vi "VariablesToString_Array.vi"(3 "Format":string="%0.2f", 4 "Terminate?":bool=TRUE, 5 "ValueIn":dbl[](array[numeric]), 6 "FieldName":string, 7 "Type":enum16{"Normal", "Matlab"}(ring)) -> (1 "StringOut":string)   [LabVIEW 2013]
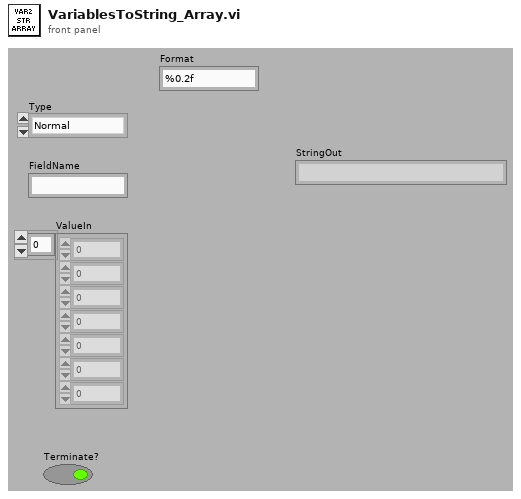
[diagram p1: front panel]
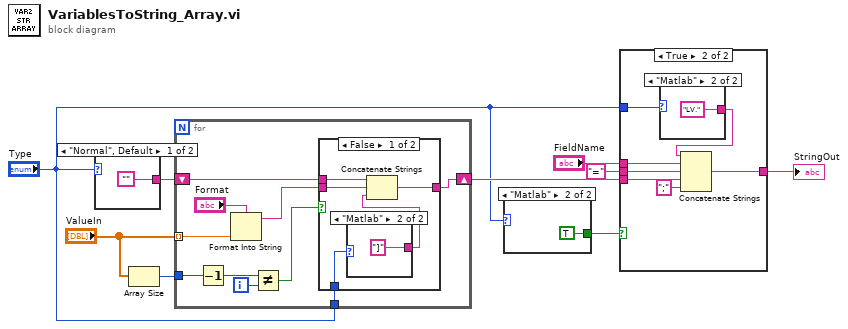
[diagram p0: block diagram]
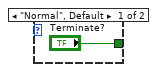
[diagram p2: hidden frame]
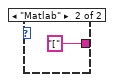
[diagram p3: hidden frame]
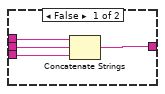
[diagram p4: hidden frame]
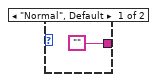
[diagram p5: hidden frame]
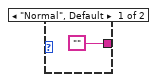
[diagram p6: hidden frame]
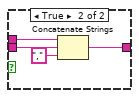
[diagram p7: hidden frame]
diagram:
  n1 = case shown="\"Normal\", Default" "Type" {
    tunnel: ["" "["] -> w7
    frame "Normal", Default {
    }
    frame "Matlab" {
    }
  }
  n2 = Array Size(array="ValueIn") -> (size(s)=w9:i32)
  n3 = for {
    tunnel: "ValueIn" -> [w21] mode=indexing
    shift-right: [w20] -> w4
    shift-left: w7 -> [w19]
    tunnel: w9 -> [w17]
    tunnel: "Type" -> [w12]
    i -> [w15]
    n4 = Decrement(x=w17) -> (x-1=w16:i32)
    n5 = Format Into String(format string="Format", w21) -> (resulting string=w18:string)  [unwired: 2 in, 1 out]
    n6 = Not Equal?(x=w16, y=w15) -> (x != y?=w14:bool)
    n7 = case shown="False" w14 {
      tunnel: [w24 w32] -> w20
      tunnel: w19 -> [w26 w31]
      tunnel: w18 -> [w25 w30]
      tunnel: w12 -> [w23 _]
      frame False {
        n8 = case shown="\"Matlab\"" w23 {
          tunnel: ["" "]"] -> w22
          frame "Normal", Default {
          }
          frame "Matlab" {
          }
        }
        n9 = Concatenate Strings(w26, w25, w22) -> (w24:string)
      }
      frame True {
        n10 = Concatenate Strings(w31, w30, "," ("string")) -> (w32:string)
      }
    }
  }
  n11 = case shown="\"Matlab\"" "Type" {
    tunnel: ["Terminate?" TRUE ("Terminate?")] -> w2
    frame "Normal", Default {
    }
    frame "Matlab" {
    }
  }
  n12 = case shown="True" w2 {
    tunnel: "FieldName" -> [w38 w45]
    tunnel: "=" ("string") -> [w37 w44]
    tunnel: w4 -> [w36 w43]
    tunnel: [w35 w41] -> w3
    tunnel: "Type" -> [_ w39]
    frame False {
      n13 = Concatenate Strings(w38, w37, w36) -> (w35:string)
    }
    frame True {
      n14 = case shown="\"Matlab\"" w39 {
        tunnel: ["" "LV."] -> w40
        frame "Normal", Default {
        }
        frame "Matlab" {
        }
      }
      n15 = Concatenate Strings(w40, w45, w44, w43, ";" ("string")) -> (w41:string)
    }
  }
  "StringOut" <- w3
